vi "Initialise.vi"(11 "Screen Dimensions":T1) -> (3 "Pixel Data out":u32[][](array[numeric]))   [LabVIEW 2022 SP3, in "Raster.lvlib"]
uses:
  Raster.lvlib
  Rectangle Dimensions.ctl
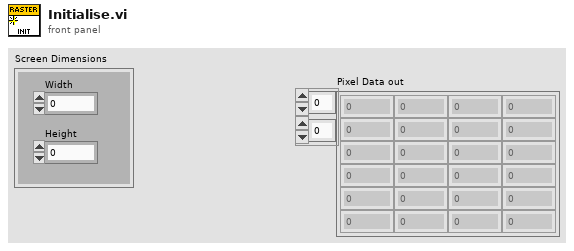
[diagram p1: front panel]
types:
  T1 = typedef "Raster.lvlib/Rectangle Dimensions.ctl" = cluster{"Width":u32, "Height":u32}
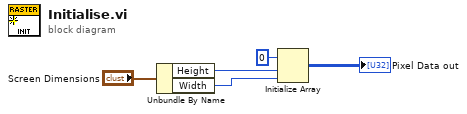
[diagram p0: block diagram]
diagram:
  n1 = Unbundle By Name("Screen Dimensions") -> ("Height"=w2:u32, "Width"=w3:u32)
  n2 = Initialize Array(u32 0 ("element"), w2, w3) -> (→"Pixel Data out":u32[][])
